vi "Load Settings.vi"(7 "Path":path, 8 "error in (no error)":errorcluster, 10 "Reader Object":refnum<class>, 11 "Scanner Object":refnum<class>) -> (0 "error out":errorcluster)   [LabVIEW 2015, in "File IO.lvclass"]
uses:
  File IO/File IO.lvclass
  Scanners/Scanner/Write Range UI.vi
  File IO/Setup UI.vi
  <vilib>/Utility/xml.llb/Read From XML File(string).vi
  Scanners/Scanner/Scanner.lvclass
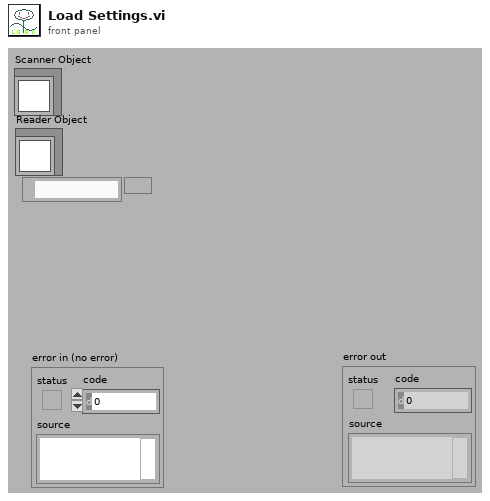
[diagram p1: front panel]
types:
  T1 = cluster{"input cluster":cluster{i32[][], string[]}, "input cluster":cluster{i32[][], string[]}, "input cluster":cluster{i32[][], string[]}, "input cluster":cluster{i32[][], string[]}}
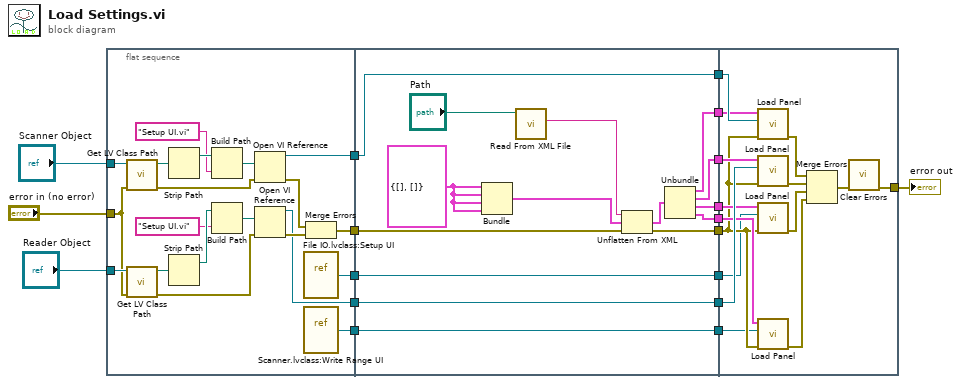
[diagram p0: block diagram]
diagram:
  n1 = flat-sequence {
    tunnel: "Scanner Object" -> [w28]
    tunnel: "Reader Object" -> [w27]
    tunnel: "error in (no error)" -> [w26]
    tunnel: [w23] -> w17
    tunnel: [w22] -> w16
    tunnel: [w21] -> w13
    tunnel: [w20] -> w3
    tunnel: [w19] -> w1
    tunnel: w17 -> [w48]
    tunnel: w16 -> [w47]
    tunnel: [w47] -> w15
    tunnel: [w46] -> w14
    tunnel: w13 -> [w45]
    tunnel: [w45] -> w12
    tunnel: [w44] -> w11
    tunnel: [w43] -> w10
    tunnel: [w42] -> w9
    tunnel: [w41] -> w8
    tunnel: [w40] -> w4
    tunnel: w3 -> [w40]
    tunnel: [w39] -> w2
    tunnel: w1 -> [w39]
    tunnel: w15 -> [w68]
    tunnel: w14 -> [w67]
    tunnel: w12 -> [w66]
    tunnel: w11 -> [w65]
    tunnel: w10 -> [w64]
    tunnel: w9 -> [w63]
    tunnel: w8 -> [w62]
    tunnel: [w56] -> w7
    tunnel: w4 -> [w55]
    tunnel: w2 -> [w54]
    frame #0 {
      n2 = call <vilib>:"Get LV Class Path.vi"("error in (no error)"=w26, "object"=w28) -> ("error out"=w34:errorcluster, "class path"=w38:path)  [unwired: 8 out]
      n3 = call <vilib>:"Get LV Class Path.vi"("error in (no error)"=w26, "object"=w27) -> ("error out"=w29:errorcluster, "class path"=w33:path)  [unwired: 8 out]
      n4 = Strip Path(path=w38) -> (stripped path=w37:path)  [unwired: 1 out]
      n5 = Strip Path(path=w33) -> (stripped path=w32:path)  [unwired: 1 out]
      n6 = Build Path(base path=w37, name or relative path="Setup UI.vi") -> (appended path=w35:path)
      n7 = Build Path(base path=w32, name or relative path="Setup UI.vi") -> (appended path=w30:path)
      n8 = Open VI Reference(vi path=w35, error in (no error)=w34) -> (vi reference=w22:refnum<vi>, error out=w25:errorcluster)  [unwired: 4 out]
      n9 = Open VI Reference(vi path=w30, error in (no error)=w29) -> (vi reference=w21:refnum<vi>, error out=w24:errorcluster)  [unwired: 4 out]
      n10 = vi-ref "File IO.lvclass:Setup UI.vi"() -> (w20:refnum<vi>)
      n11 = vi-ref "Scanner.lvclass:Write Range UI.vi"() -> (w19:refnum<vi>)
      n12 = Merge Errors(w25, w24) -> (w23:errorcluster)
    }
    frame #1 {
      w50 = cluster{i32[][], string[]} {[], []} ("input cluster")
      n13 = Bundle("input cluster"=w50, "input cluster"=w50, "input cluster"=w50, "input cluster"=w50) -> (w49:T1)  [unwired: 1 in]
      n14 = call-poly <vilib>:"Read From XML File.vi"("XML File Path"="Path") -> ("XML Elements"=w51:string)  [unwired: 8 in, 2 out]
      n15 = Unflatten From XML(xml string=w51, type=w49, error in (no error)=w48) -> (value=w52:T1, error out=w41:errorcluster)
      n16 = Unbundle(w52) -> ("input cluster"=w46:cluster{i32[][], string[]}, "input cluster"=w44:cluster{i32[][], string[]}, "input cluster"=w43:cluster{i32[][], string[]}, "input cluster"=w42:cluster{i32[][], string[]})
    }
    frame #2 {
      n17 = call "Load Panel.vi"("error in (no error)"=w62, "vi reference"=w68, "value"=w67) -> ("error out"=w60:errorcluster)  [unwired: 8 in]
      n18 = call "Load Panel.vi"("error in (no error)"=w62, "vi reference"=w66, "value"=w65) -> ("error out"=w59:errorcluster)  [unwired: 8 in]
      n19 = call "Load Panel.vi"("error in (no error)"=w62, "vi reference"=w55, "value"=w64) -> ("error out"=w58:errorcluster)  [unwired: 8 in]
      n20 = call "Load Panel.vi"("error in (no error)"=w62, "vi reference"=w54, "value"=w63) -> ("error out"=w57:errorcluster)  [unwired: 8 in]
      n21 = Merge Errors(w60, w59, w58, w57) -> (w61:errorcluster)
      n22 = call <vilib>:"Clear Errors.vi"("error in (no error)"=w61) -> ("error out"=w56:errorcluster)  [unwired: 5 in, 1 out]
    }
  }
  "error out" <- w7
